vi "Dependency Migration Main.vi"(0 "LibraryRefnum":refnum<vi>, 5 "Project:Open":refnum<vi>, 7 "SourceModulePath":path=path "D:/Magnum_Nexus/Dependency Migration/SampleModules/MeasurementProject/Flat.vi", 11 "error in (no error)":errorcluster) -> (4 "InstrContaining":path[](array[path]), 15 "error out":errorcluster)   [LabVIEW 2021, in "Migrator.lvlib"]
uses:
  Migrator.lvlib
  Migrator Reusables/Migrator Reusables.lvlib
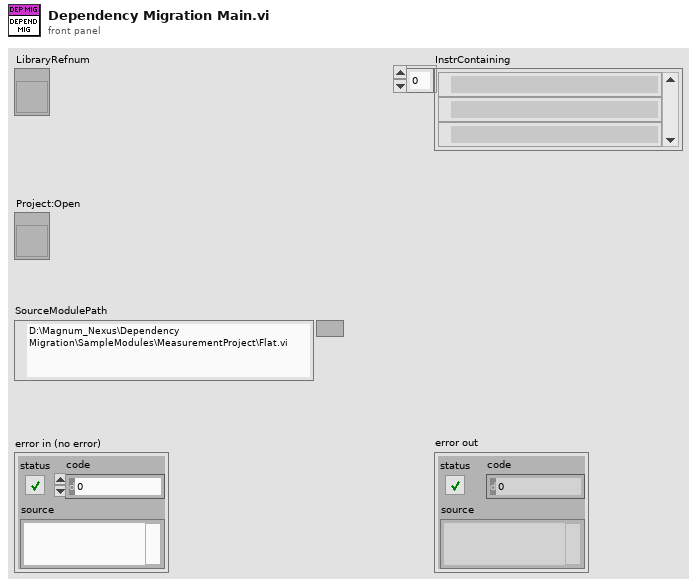
[diagram p1: front panel]
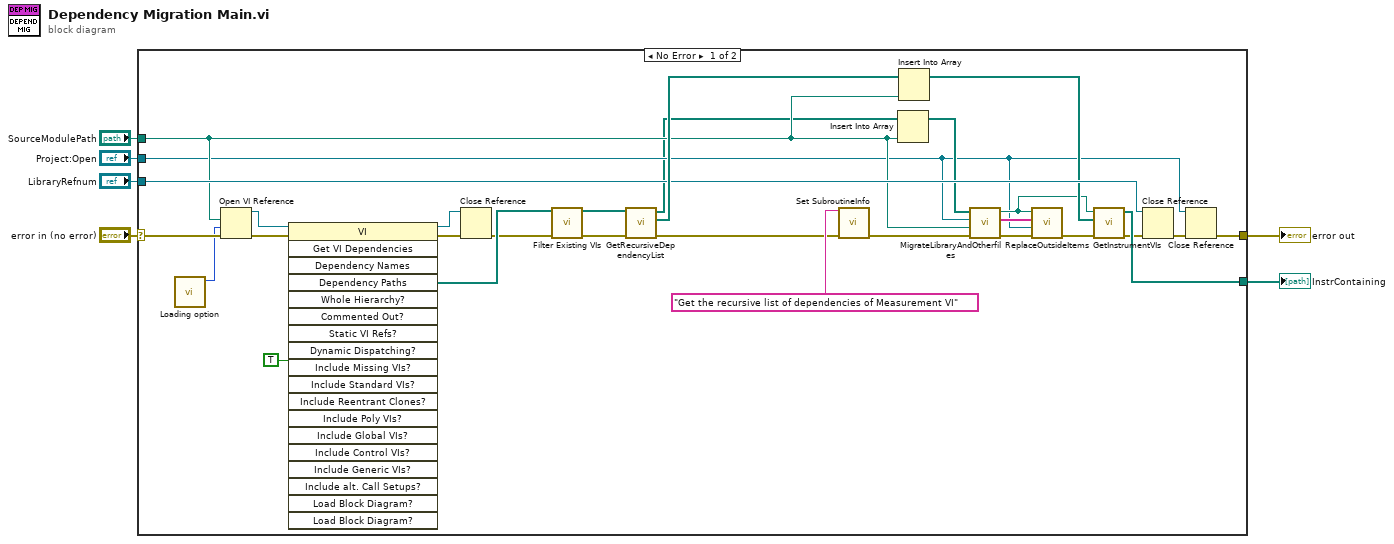
[diagram p0: block diagram]
diagram:
  n1 = case shown="No Error" "error in (no error)" {
    selector: "error in (no error)" -> [w26 w36]
    tunnel: "LibraryRefnum" -> [w29 _]
    tunnel: [w27 _] -> w5
    tunnel: [w23 w36] -> w3
    tunnel: "SourceModulePath" -> [w17 _]
    tunnel: "Project:Open" -> [w16 _]
    frame No Error {
      n2 = call "Loading option.vi"() -> ("options"=w15:i32)  [unwired: 11 in]
      n3 = Open VI Reference(vi path=w17, options=w15, error in (no error)=w26) -> (vi reference=w34:refnum<vi>, error out=w35:errorcluster)  [unwired: 3 in]
      n4 = invoke class="VI" method="Get VI Dependencies"(reference=w34, error in=w35, "Include Missing VIs?"=TRUE ("Include Missing Items?")) -> (reference out=w30:refnum<vi>, error out=w31:errorcluster, "Dependency Paths"=w10:path[])  [unwired: 16 in, 16 out]
      n5 = Close Reference(reference=w30, error in (no error)=w31) -> (error out=w8:errorcluster)
      n6 = call "Filter Existing VIs.vi"("Dependency Path"=w10, "error in (no error)"=w8) -> ("Valid Dep Path"=w9:path[], "error out"=w7:errorcluster)  [unwired: 12 in]
      n7 = call "GetRecursiveDependencyList.vi"("error in (no error)"=w7, "Dependency Paths"=w9) -> ("error out"=w11:errorcluster, "InstrContaining"=w33:path[], "Array"=w12:path[])  [unwired: 7 in]
      n8 = call "Set SubroutineInfo.vi"("Subroutine In"="Get the recursive list of dependencies of Measurement VI", "error in (no error)"=w11) -> ("error out"=w14:errorcluster)  [unwired: 13 in]
      n9 = Insert Into Array(array=w12, new element=w17) -> (w22:path[])  [unwired: 1 in]
      n10 = Insert Into Array(array=w33, new element=w17) -> (w28:path[])  [unwired: 1 in]
      n11 = call "MigrateLibraryAndOtherfiles.vi"("error in (no error)"=w14, "MainModulePath"=w17, "Project:Open"=w16, "DependencyList[]"=w22) -> ("error out"=w21:errorcluster, "OutsideVIs"=w18:string[], "DestinationDirectory"=w19:path)  [unwired: 5 in]
      n12 = call "ReplaceOutsideItems.vi"("error in (no error)"=w21, "Project:Open"=w16, "OutsideVIs"=w18, "DestinationDirectory"=w19) -> ("error out"=w20:errorcluster)  [unwired: 7 in]
      n13 = call "GetInstrumentVIs.vi"("error in (no error)"=w20, "InstrContaining"=w28, "DestinationDirectory"=w19) -> ("error out"=w24:errorcluster, "InstrContainingVI[]"=w27:path[])  [unwired: 7 in]
      n14 = Close Reference(reference=w29, error in (no error)=w24) -> (error out=w25:errorcluster)
      n15 = Close Reference(reference=w16, error in (no error)=w25) -> (error out=w23:errorcluster)
    }
    frame Error {
    }
  }
  "error out" <- w3
  "InstrContaining" <- w5
